vi "Close_DSP.vi"(8 "error in (no error)":errorcluster caption="에러 입력(에러 없음)", 11 "VISA resource name":refnum<visa-resource-name>) -> (0 "error out":errorcluster)   [LabVIEW 2019]
uses:
  cbb21dde-4b10-46cf-8286-ae54b4875113.vi
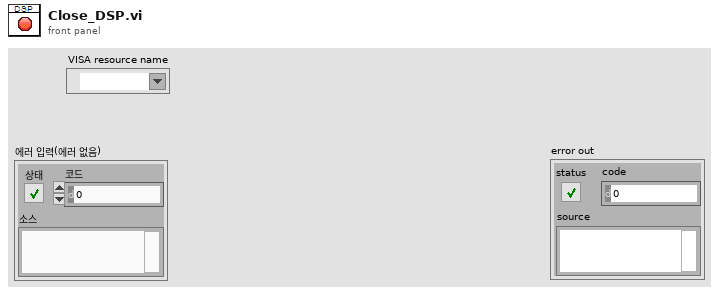
[diagram p1: front panel]
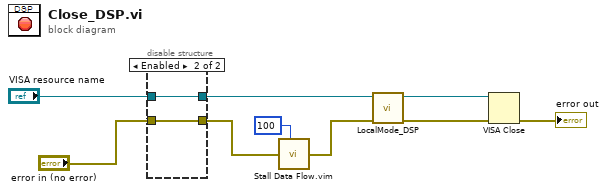
[diagram p0: block diagram]
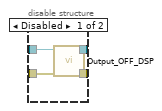
[diagram p2: hidden frame]
diagram:
  n1 = disable-structure shown="Enabled" {
    disable-tunnel: "VISA resource name" -> [w13 w15]
    disable-tunnel: "error in (no error)" -> [w12 w14]
    disable-tunnel: [w11 w14] -> w5
    disable-tunnel: [w10 w15] -> w3
    frame Disabled {
      n2 = call "Output_OFF_DSP.vi"("error in"=w12, "VISA"=w13) -> ("error out"=w11:errorcluster, "VISA2"=w10:refnum<visa-resource-name>)  [unwired: 8 in]
    }
    frame Enabled {
    }
  }
  n3 = call "Stall Data Flow.vim"("value in"=w5, "milliseconds to wait"=u32 100) -> ("value out"=w4:errorcluster)  [unwired: 1 out]
  n4 = call "LocalMode_DSP.vi"("error in (no error)"=w4, "VISA resource name"=w3) -> ("error out"=w1:errorcluster, "VISA resource name Out"=w2:refnum<visa-resource-name>)  [unwired: 8 in]
  n5 = VISA Close(VISA resource name=w2, error in (no error)=w1) -> (error out=→"error out":errorcluster)
